vi "MISSION_REQUEST.vi"(0 "sequence":u16=6, 5 "target_system":u8=6, 7 "target_component":u8=8) -> (4 "MAVLink Message":u8[](array[numeric]))   [LabVIEW 2014]
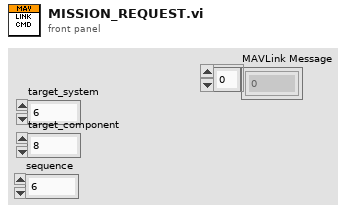
[diagram p1: front panel]
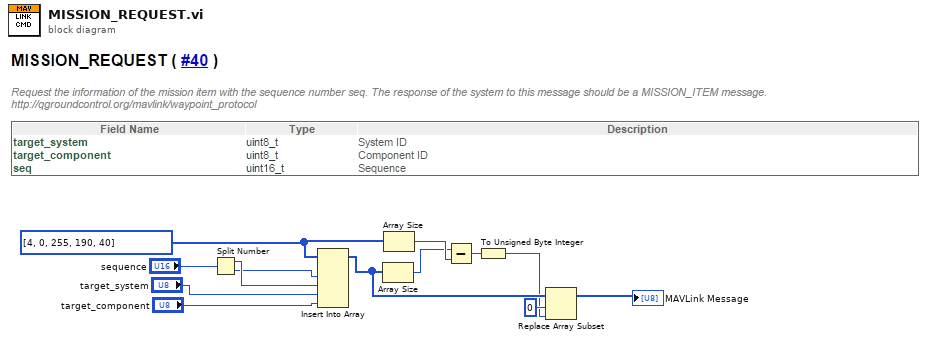
[diagram p0: block diagram]
diagram:
  w13 = u8[] [4, 0, 255, 190, 40]
  n1 = Split Number(x="sequence") -> (hi(x)=w2:u8, lo(x)=w1:u8)
  n2 = Insert Into Array(array=w13, new element #1=w1, new element #2=w2, new element #3="target_system", new element #4="target_component") -> (w9:u8[])  [unwired: 1 in]
  n3 = Array Size(array=w9) -> (size(s)=w11:i32)
  n4 = Array Size(array=w13) -> (size(s)=w12:i32)
  n5 = Subtract(x=w11, y=w12) -> (x-y=w10:i32)
  n6 = To Unsigned Byte Integer(number=w10) -> (unsigned 8bit integer=w7:u8)
  n7 = Replace Array Subset(array=w9, new element=w7, index=0) -> (→"MAVLink Message":u8[])
